vi "Rename gRPC Server Class.vi"(4 "new class name":string, 6 "old class name":string, 8 "error in (no error)":errorcluster, 10 "library name":string, 11 "path to project":path) -> (0 "error out":errorcluster)   [LabVIEW 2020]
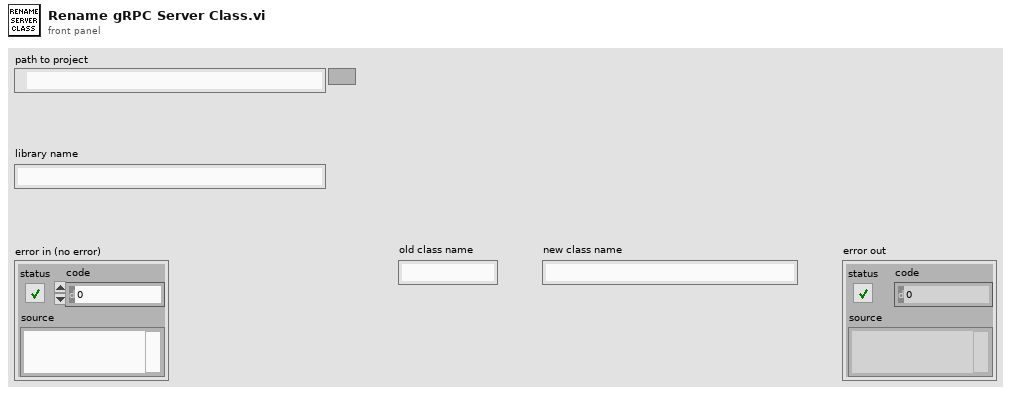
[diagram p1: front panel]
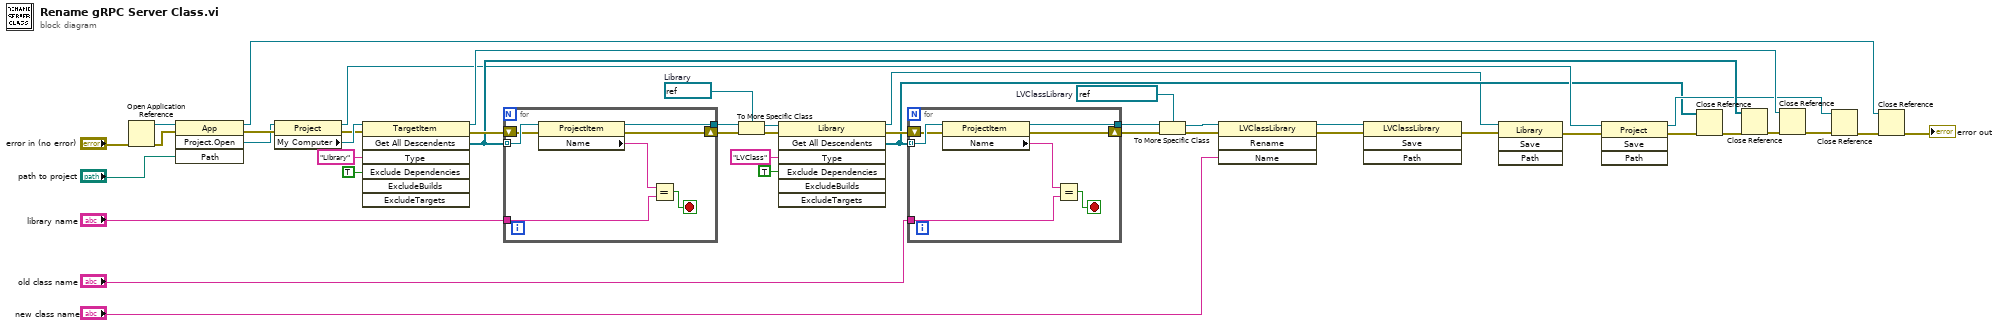
[diagram p0: block diagram]
diagram:
  w20 = refnum<vi> refnum  # Library
  w26 = refnum<vi> refnum  # LVClassLibrary
  n1 = Open Application Reference(8:"error in (no error)") -> (0:w38:errorcluster, 3:w37:refnum<vi>)  [unwired: 3 in]
  n2 = invoke class="App" method="Project.Open"(reference=w37, error in=w38, "Path"="path to project") -> (reference out=w1:refnum<vi>, error out=w41:errorcluster, "Project:Open"=w40:refnum<vi>)  [unwired: 1 in, 1 out]
  n3 = property class="Project"(reference=w40, error in=w41) -> (reference out=w17:refnum<vi>, error out=w42:errorcluster, "My Computer"=w43:refnum<vi>)
  n4 = invoke class="TargetItem" method="Get All Descendents"(reference=w43, error in=w42, "Type"="Library", "Exclude Dependencies"=TRUE ("ExcludeDependencies")) -> (reference out=w18:refnum<vi>, error out=w33:errorcluster, "All Descendents"=w25:refnum<vi>[])  [unwired: 3 in, 4 out]
  n5 = for {
    tunnel: w25 -> [w51] mode=indexing
    tunnel: "library name" -> [w49]
    shift-right: [w46] -> w24
    shift-left: w33 -> [w47]
    tunnel: [w45] -> w22
    stop <- w48 stop-if-true
    n6 = property class="ProjectItem"(reference=w51, error in=w47) -> (reference out=w45:refnum<vi>, error out=w46:errorcluster, "Name"=w50:string)
    n7 = Equal?(x=w50, y=w49) -> (x = y?=w48:bool)
  }
  n8 = To More Specific Class(target class=w20, reference=w22, error in=w24) -> (specific class reference=w21:refnum<vi>, error out=w23:errorcluster)
  n9 = invoke class="Library" method="Get All Descendents"(reference=w21, error in=w23, "Type"="LVClass", "Exclude Dependencies"=TRUE ("ExcludeDependencies")) -> (reference out=w2:refnum<vi>, error out=w30:errorcluster, "All Descendents"=w11:refnum<vi>[])  [unwired: 3 in, 4 out]
  n10 = for {
    tunnel: w11 -> [w58] mode=indexing
    tunnel: "old class name" -> [w57]
    shift-right: [w55] -> w28
    shift-left: w30 -> [w56]
    tunnel: [w54] -> w27
    stop <- w52 stop-if-true
    n11 = property class="ProjectItem"(reference=w58, error in=w56) -> (reference out=w54:refnum<vi>, error out=w55:errorcluster, "Name"=w53:string)
    n12 = Equal?(x=w53, y=w57) -> (x = y?=w52:bool)
  }
  n13 = To More Specific Class(target class=w26, reference=w27, error in=w28) -> (specific class reference=w8:refnum<vi>, error out=w7:errorcluster)
  n14 = invoke class="LVClassLibrary" method="Rename"(reference=w8, error in=w7, "Name"="new class name") -> (reference out=w5:refnum<vi>, error out=w4:errorcluster)  [unwired: 1 in, 2 out]
  n15 = invoke class="LVClassLibrary" method="Save"(reference=w5, error in=w4) -> (error out=w3:errorcluster)  [unwired: 2 in, 3 out]
  n16 = invoke class="Library" method="Save"(reference=w2, error in=w3) -> (error out=w13:errorcluster)  [unwired: 2 in, 3 out]
  n17 = invoke class="Project" method="Save"(reference=w17, error in=w13) -> (reference out=w16:refnum<vi>, error out=w12:errorcluster)  [unwired: 2 in, 2 out]
  n18 = Close Reference(reference=w11, error in (no error)=w12) -> (error out=w10:errorcluster)
  n19 = Close Reference(reference=w25, error in (no error)=w10) -> (error out=w19:errorcluster)
  n20 = Close Reference(reference=w18, error in (no error)=w19) -> (error out=w9:errorcluster)
  n21 = Close Reference(reference=w16, error in (no error)=w9) -> (error out=w15:errorcluster)
  n22 = Close Reference(reference=w1, error in (no error)=w15) -> (error out=→"error out":errorcluster)
